vi "Open.vi"(6 "Length Parameter (0, 4, Big, 0)":T1={"Byte Offset"=0, "Byte Size"=4, "Endian"=enum."Big", "Add"=0}, 8 "error in (no error)":errorcluster, 9 "Create if not found? (T)":bool=TRUE, 10 "Ports (5123, 5123)":cluster{"Cmd Port":u16, "Tlm Port":u16}={"Cmd Port"=5123, "Tlm Port"=5123}, 11 "App ID in":u16) -> (0 "error out":errorcluster, 1 "Created New?":bool, 3 "App ID out":u16)   [LabVIEW 2018, in "TCPServer.lvlib"]
uses:
  TCPServer.lvlib
  TypeDefs/App.ctl
  SubVIs/Daemon.vi
  TypeDefs/Connection.ctl
  <vilib>/ErrorRing/Error Ring.xnode
  <vilib>/Utility/error.llb/Error Cluster From Error Code.vi
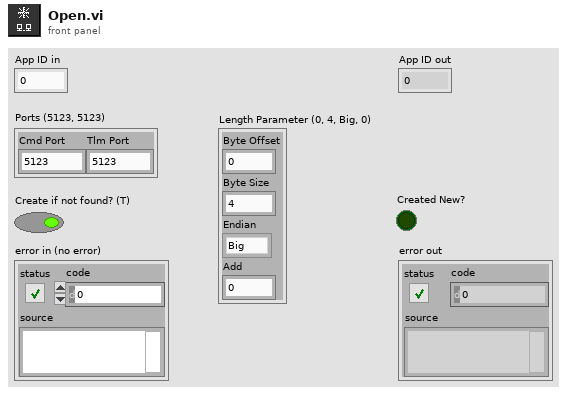
[diagram p1: front panel]
types:
  T1 = cluster{"Byte Offset":i32, "Byte Size":i32, "Endian":enum8{"Big", "Little"}, "Add":i32}
  T2 = typedef "TCPServer.lvlib/App.ctl" = cluster{"Stack":refnum<queue>, "Cmd":cluster{"Conn":refnum<data-value>, "Daemon":refnum<vi>, "Counter":refnum<data-value>}, "Tlm":cluster{"Conn":refnum<data-value>, "Daemon":refnum<vi>, "Counter":refnum<data-value>}}
  T3 = cluster{"Conn":refnum<data-value>, "Daemon":refnum<vi>, "Counter":refnum<data-value>}
  T4 = typedef "TCPServer.lvlib/Connection.ctl" = cluster{"Tcp":refnum<k5>, "Server Port":u16, "Server Port Type":enum8{"CMD", "TLM", "BOTH"}, "Client IP":string, "Client Port":u16}
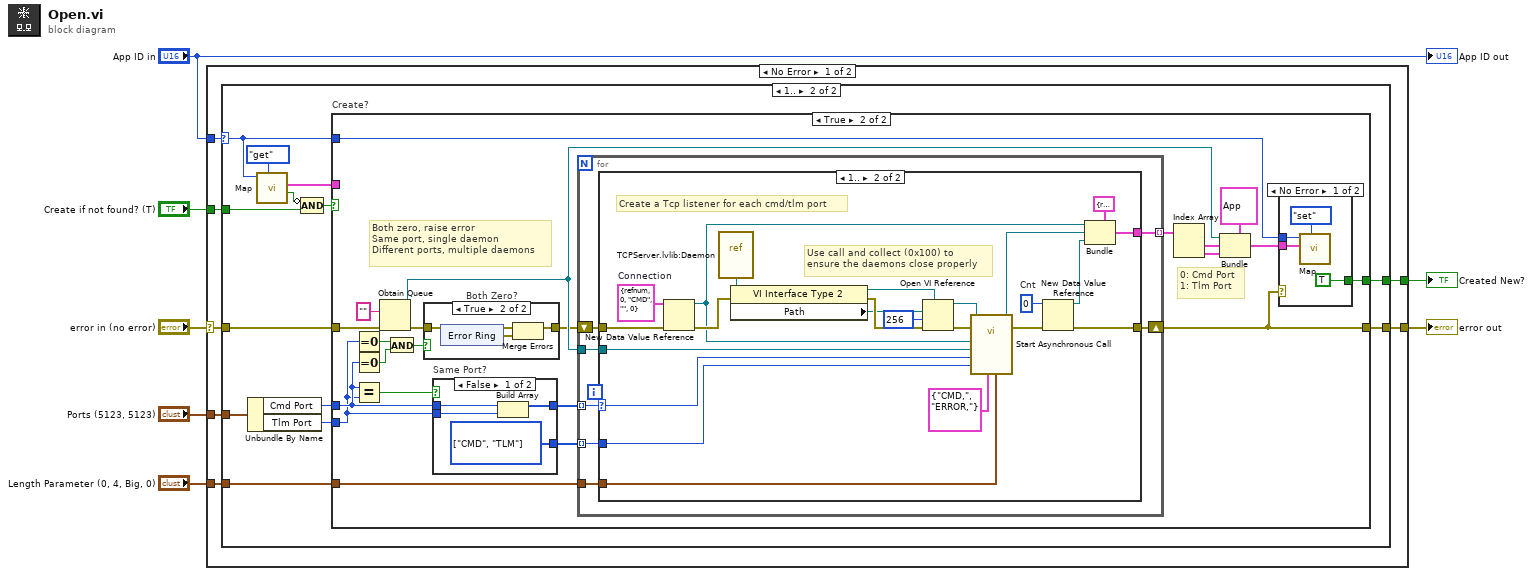
[diagram p0: block diagram]
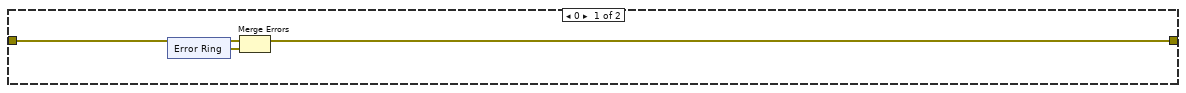
[diagram p2: hidden frame]
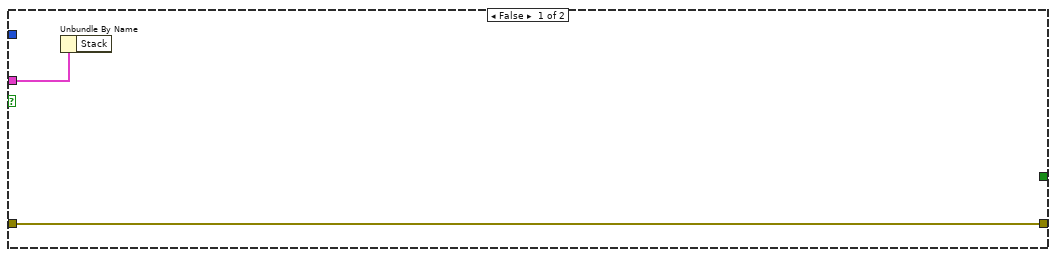
[diagram p3: hidden frame]
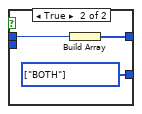
[diagram p5: hidden frame]
diagram:
  n1 = case shown="No Error" "error in (no error)" {
    selector: "error in (no error)" -> [w12 w111]
    tunnel: "App ID in" -> [w11 _]
    tunnel: "Ports (5123, 5123)" -> [w9 _]
    tunnel: [w14 w111] -> w6
    tunnel: "Length Parameter (0, 4, Big, 0)" -> [w13 _]
    tunnel: "Create if not found? (T)" -> [w10 _]
    tunnel: [w8 _] -> w2
    frame No Error {
      n2 = case shown="1.." w11 {
        selector: w11 -> [_ w31]
        tunnel: [w16 w35] -> w14
        tunnel: w13 -> [_ w34]
        tunnel: w12 -> [w15 w33]
        tunnel: w10 -> [_ w29]
        tunnel: w9 -> [_ w27]
        tunnel: [_ w24] -> w8
        frame 0 {
          n3 = xnode "Error Ring"() -> ("error out"=w17:errorcluster)
          n4 = Merge Errors(w15, w17) -> (w16:errorcluster)
        }
        frame 1.. {
          n5 = Unbundle By Name(w27) -> ("Cmd Port"=w26:u16, "Tlm Port"=w25:u16)
          n6 = call "Map.vi"("Action"=enum8{"noop", "get", "set", "pop"}."get", "App ID in"=w31) -> ("Found?"=w30:bool, "App out"=w23:T2)  [unwired: 7 in, 1 out]
          n7 = Compound Arithmetic op=AND(invert w30, w29) -> (w28:bool)
          n8 = case "Create?" shown="True" w28 {
            tunnel: [w37 w39] -> w35
            tunnel: w34 -> [_ w58]
            tunnel: w33 -> [w37 w45]
            tunnel: w31 -> [_ w42]
            tunnel: w26 -> [_ w41]
            tunnel: w25 -> [_ w40]
            tunnel: [_ w38] -> w24
            tunnel: w23 -> [w36 _]
            frame False {
              n9 = Unbundle By Name(w36) -> ()  [unwired: 1 out]
            }
            frame True {
              # "0: Cmd Port\n1: Tlm Port"
              # "Both zero, raise error\nSame port, single daemon\nDifferent ports, multiple daemons"
              n10 = Equal To 0?(x=w40) -> (x = 0?=w57:bool)
              n11 = Equal To 0?(x=w41) -> (x = 0?=w56:bool)
              n12 = Equal?(x=w41, y=w40) -> (x = y?=w54:bool)
              n13 = Obtain Queue(element data type="", error in (no error)=w45) -> (queue out=w59:refnum<queue>, error out=w44:errorcluster)  [unwired: 3 in, 1 out]
              n14 = And(x=w57, y=w56) -> (x .and. y?=w55:bool)
              n15 = case "Both Zero?" shown="True" w55 {
                tunnel: w44 -> [w71 w74]
                tunnel: [w71 w73] -> w43
                frame False {
                }
                frame True {
                  n16 = xnode "Error Ring"() -> ("error out"=w72:errorcluster)
                  n17 = Merge Errors(w74, w72) -> (w73:errorcluster)
                }
              }
              n18 = case "Same Port?" shown="False" w54 {
                tunnel: [w67 w69] -> w53
                tunnel: w41 -> [w66 w70]
                tunnel: w40 -> [w65 _]
                tunnel: [w64 w68] -> w52
                frame False {
                  w64 = enum8{"CMD", "TLM", "BOTH"}[] [enum."CMD", enum."TLM"] items=["CMD", "TLM", "BOTH"]
                  n19 = Build Array(w66, w65) -> (w67:u16[])
                }
                frame True {
                  w68 = enum8{"CMD", "TLM", "BOTH"}[] [enum."BOTH"] items=["CMD", "TLM", "BOTH"]
                  n20 = Build Array(w70) -> (w69:u16[])
                }
              }
              n21 = for {
                tunnel: w59 -> [w86]
                tunnel: w53 -> [w85] mode=indexing
                tunnel: w52 -> [w84] mode=indexing
                shift-right: [w80] -> w39
                shift-left: w43 -> [w83]
                tunnel: w58 -> [w82]
                tunnel: [w81] -> w50 mode=indexing
                n22 = case shown="1.." w85 {
                  selector: w85 -> [_ w102]
                  tunnel: w86 -> [_ w103]
                  tunnel: w84 -> [_ w101]
                  tunnel: w83 -> [w87 w100]
                  tunnel: w82 -> [_ w97]
                  tunnel: [_ w94] -> w81
                  tunnel: [w87 w90] -> w80
                  frame 0 {
                  }
                  frame 1.. {
                    w93 = u16 0  # Cnt
                    w98 = T4 {"Tcp"=refnum, "Server Port"=0, "Server Port Type"=enum."CMD", "Client IP"="", "Client Port"=0}  # Connection
                    # "Use call and collect (0x100) to\nensure the daemons close properly"
                    # "Create a Tcp listener for each cmd/tlm port"
                    n23 = New Data Value Reference(data value=w98, error in=w100) -> (data value reference=w96:refnum<data-value>, error out=w99:errorcluster)
                    n24 = vi-ref "TCPServer.lvlib:Daemon.vi"() -> (w108:refnum<vi>)
                    n25 = property class="VI Interface Type 2"(reference=w108, error in=w99) -> (reference out=w104:refnum<vi>, error out=w109:errorcluster, "Path"=w107:path)
                    n26 = Open VI Reference(type specifier VI Refnum (for type only)=w104, vi path=w107, options=256, error in (no error)=w109) -> (vi reference=w105:refnum<vi>, error out=w110:errorcluster)  [unwired: 2 in]
                    n27 = call-by-ref "Start Asynchronous Call"(reference=w105, error in=w110, "Length"=w97, "Interrupts"=cluster{"Cmd":string, "Error":string} {"Cmd"="CMD,", "Error"="ERROR,"} ("Interrupts (\"CMD,\", \"ERROR,\")"), "Port Type"=w101, "Port"=w102, "Target Queue"=w103, "Connection"=w96) -> (reference out=w95:refnum<vi>, error out=w92:errorcluster)  [unwired: 6 in]
                    n28 = New Data Value Reference(data value=w93, error in=w92) -> (data value reference=w91:refnum<data-value>, error out=w90:errorcluster)
                    n29 = Bundle(cluster=T3 {"Conn"=refnum, "Daemon"=refnum, "Counter"=refnum} ("Cmd"), "Conn"=w96, "Daemon"=w95, "Counter"=w91) -> (w94:T3)
                  }
                }
              }
              n30 = Index Array(array=w50) -> (element #1=w48:T3, element #2=w47:T3)  [unwired: 2 in]
              n31 = Bundle(cluster=T2 {"Stack"=refnum, "Cmd"={"Conn"=refnum, "Daemon"=refnum, "Counter"=refnum}, "Tlm"={"Conn"=refnum, "Daemon"=refnum, "Counter"=refnum}} ("ASIST"), "Stack"=w59, "Cmd"=w48, "Tlm"=w47) -> (w46:T2)
              n32 = case shown="No Error" w39 {
                tunnel: w46 -> [w62 _]
                tunnel: w42 -> [w61 _]
                tunnel: [TRUE _] -> w38
                frame No Error {
                  n33 = call "Map.vi"("Action"=enum8{"noop", "get", "set", "pop"}."set", "App in"=w62, "App ID in"=w61) -> ()  [unwired: 6 in, 3 out]
                }
                frame Error {
                }
              }
            }
          }
        }
      }
    }
    frame Error {
    }
  }
  "error out" <- w6
  "Created New?" <- w2
  "App ID out" <- "App ID in"
